vi "Read.vi"(7 "I2C Channel (0)":u8, 8 "Error In":errorcluster, 9 "Resolution":enum16{"0.5", "0.25", "0.125", "0.0625"}(ring), 10 "Slave Address":T1(ring), 11 "LINX Resource":T2) -> (0 "Error Out":errorcluster, 2 "Ambient Temperature (C)":dbl, 3 "LINX Resource":T2)   [LabVIEW 2019, in "LMH-LINX.lvlib" / "PmodTMP3.lvlib"]
doc: "Read temperature data in C from the PmodTMP3."
uses:
  <vilib>/MakerHub/LINX/Public/Sensors/Pmods/TMP3/PmodTMP3.lvlib
  <vilib>/MakerHub/LINX/Private/Type Defs/LINX Ref.ctl
  <vilib>/MakerHub/LINX/Private/Type Defs/Platform.ctl
  <vilib>/MakerHub/LINX/Private/Type Defs/Interface.ctl
  <vilib>/MakerHub/LINX/Private/Device/Type Defs/LINX Device Config.ctl
  <vilib>/MakerHub/LINX/Private/Device/Type Defs/TCP Config.ctl
  <vilib>/MakerHub/LINX/Private/Device/Type Defs/Channels.ctl
  <vilib>/MakerHub/LINX/Private/Local IO/LinxI2cWrite.vi
  <vilib>/MakerHub/LINX/Public/Utilities/Check Channel.vi
  <vilib>/MakerHub/LINX/Private/Utilties/Generate Error.vi
  <vilib>/MakerHub/LINX/LMH-LINX.lvlib
  <vilib>/MakerHub/Toolbox/LMH-Toolbox.lvlib
  <vilib>/MakerHub/LINX/Private/Device/Device.lvlib
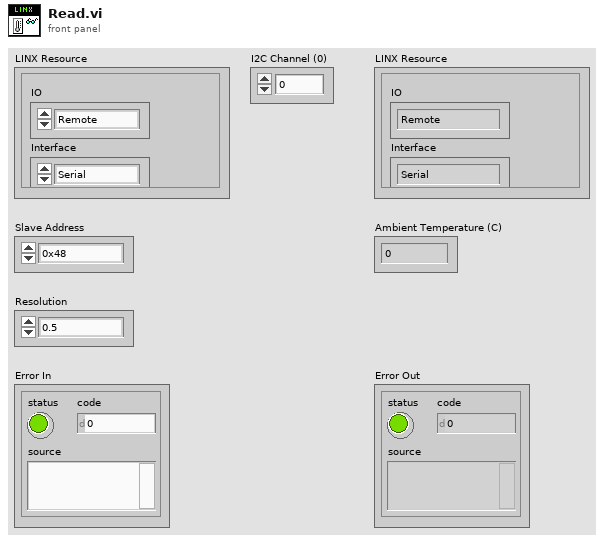
[diagram p1: front panel]
types:
  T1 = enum8{"0x48", "0x49", "0x4A", "0x4B", "0x4C", "0x4D", "0x4E", "0x4F"}
  T2 = typedef "LMH-LINX.lvlib/LINX Ref.ctl" = cluster{"IO":T3, "Interface":T4, "LINX Device Config":T5}
  T3 = typedef "LMH-LINX.lvlib/Platform.ctl" = enum16{"Remote", "Local"}
  T4 = typedef "LMH-LINX.lvlib/Interface.ctl" = enum16{"Serial", "TCP"}
  T5 = typedef "LMH-LINX.lvlib/Device.lvlib/LINX Device Config.ctl" = cluster{"Interface":T4, "COM Port":refnum<visa-resource-name>, "TCP Configuration":T6, "Device Family":u8, "Device ID":u8, "Device Name":string, "TCP Ref":refnum<k5>, "Channels":T7}
  T6 = typedef "LMH-LINX.lvlib/Device.lvlib/TCP Config.ctl" = cluster{"IP Address":string, "Port":u16}
  T7 = typedef "LMH-LINX.lvlib/Channels.ctl" = cluster{"DI":u8[], "DO":u8[], "AI":u8[], "AO":u8[], "PWM":u8[], "QE":u8[], "UART":u8[], "I2C 2":u8[], "SPI":u8[], "CAN":u8[], "Servo":u8[], "AI Ref (V)":dbl, "AI Resolution (Bits)":u8, "AO Ref (V)":dbl, "AO Resolution (Bits)":u8}
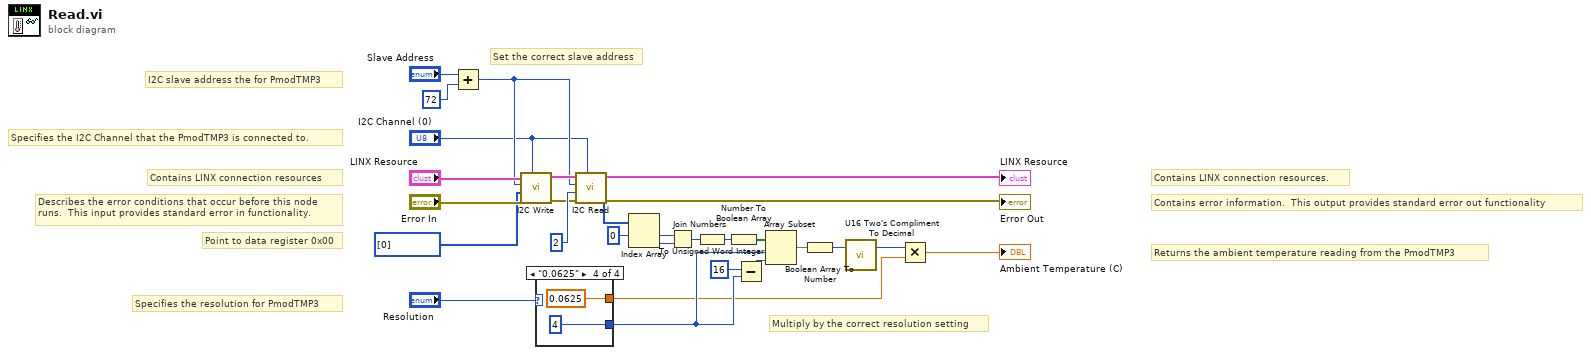
[diagram p0: block diagram]
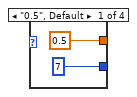
[diagram p2: hidden frame]
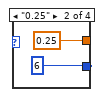
[diagram p3: hidden frame]
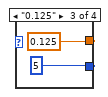
[diagram p4: hidden frame]
diagram:
  # "Returns the ambient temperature reading from the PmodTMP3"
  # "I2C slave address the for PmodTMP3"
  # "Specifies the resolution for PmodTMP3"
  # "Contains error information.  This output provides standard error out functionality"
  # "Describes the error conditions that occur before this node\nruns.  This input provides standard error in functionality."
  # "Contains LINX connection resources"
  # "Specifies the I2C Channel that the PmodTMP3 is connected to."
  # "Contains LINX connection resources."
  # "Multiply by the correct resolution setting"
  # "Point to data register 0x00"
  # "Set the correct slave address"
  n1 = Add(x="Slave Address", y=u8 72) -> (x+y=w4:u8)
  n2 = call <vilib>:"I2C Write.vi"("I2C Channel"="I2C Channel (0)", "Error In"="Error In", "Data"=u8[] [0], "I2C Slave Address (0)"=w4, "LINX Resource"="LINX Resource") -> ("Error Out"=w8:errorcluster, "LINX Resource"=w9:T2)  [unwired: 5 in]
  n3 = case shown="\"0.0625\"" "Resolution" {
    tunnel: [0.5 0.25 0.125 0.0625] -> w26
    tunnel: [7 6 5 4] -> w27
    frame "0.5", Default {
    }
    frame "0.25" {
    }
    frame "0.125" {
    }
    frame "0.0625" {
    }
  }
  n4 = call <vilib>:"I2C Read.vi"("I2C Channel"="I2C Channel (0)", "Error In"=w8, "Bytes To Read"=u8 2, "I2C Slave Address (0)"=w4, "LINX Resource"=w9) -> ("Error Out"=→"Error Out":errorcluster, "Data"=w11:u8[], "LINX Resource"=→"LINX Resource":T2)  [unwired: 4 in]
  n5 = Index Array(array=w11, index #1=0 ("index")) -> (element #1=w14:u8, element #2=w13:u8)  [unwired: 1 in]
  n6 = Join Numbers(hi=w14, lo=w13) -> ((hi.lo)=w15:u16)
  n7 = To Unsigned Word Integer(number=w15) -> (unsigned 16bit integer=w16:u16)
  n8 = Number To Boolean Array(number=w16) -> (Boolean array=w17:bool[])
  n9 = Subtract(x=16, y=w27) -> (x-y=w23:i32)
  n10 = Array Subset(array=w17, index=w27, length=w23) -> (w18:bool[])
  n11 = Boolean Array To Number(Boolean array=w18) -> (number=w19:u16)
  n12 = call <vilib>:"U16 Two's Compliment To Decimal.vi"("Two's Compliment U16"=w19) -> ("Decimal I16"=w20:i16)  [unwired: 2 in]
  n13 = Multiply(x=w20, y=w26) -> (x*y=→"Ambient Temperature (C)":dbl)
